vi "Client HTTP Download.vi"(0 "http URL":string, 5 "file path (Not A Path)":path, 7 "follow redirects (T)":bool=TRUE, 9 "Port (80)":u16=80, 11 "error in (no error)":errorcluster) -> (2 "header":string, 3 "status":i32, 4 "full document URL":string, 6 "file path out":path, 8 "file error":errorcluster, 10 "success":bool, 13 "content-type":string, 14 "content":string, 15 "error out":errorcluster)   [LabVIEW 2011]
doc: "Retrieves a document specified by <B>http URL</B> and stores it in a specified file or returns the contents as a string."
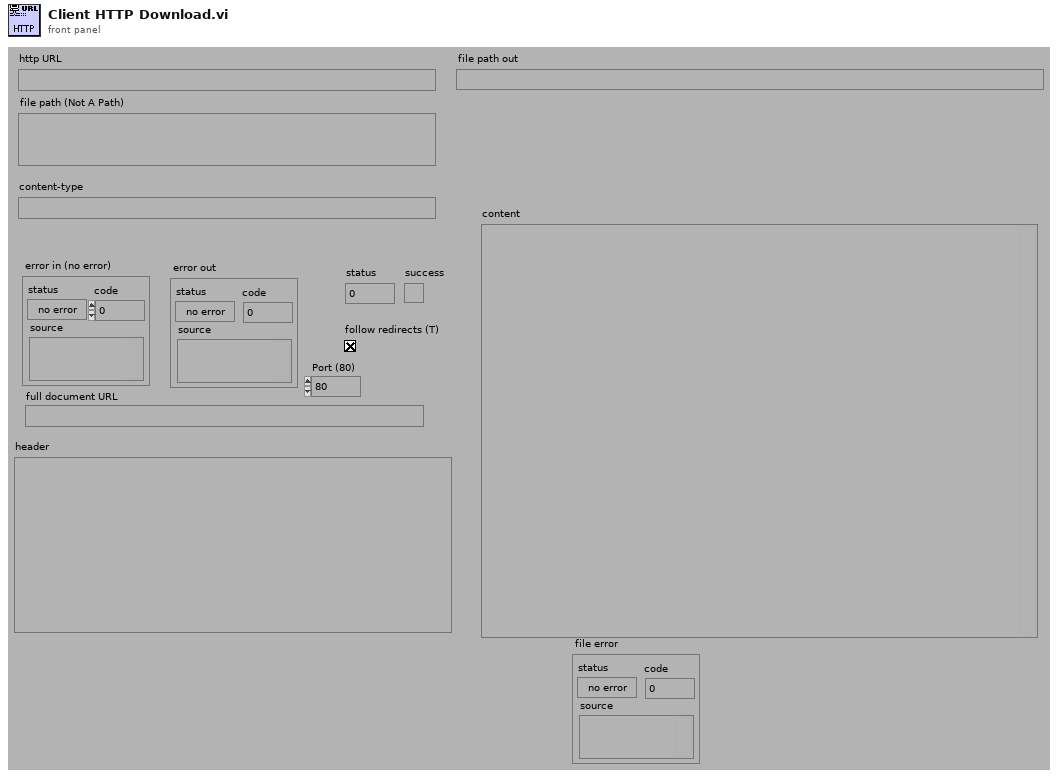
[diagram p1: front panel]
types:
  T1 = cluster{"bytes to read":i32, "timeout ms":i32, "read mode":enum16{"normal", "line", "buffered"}, "line separator":string}
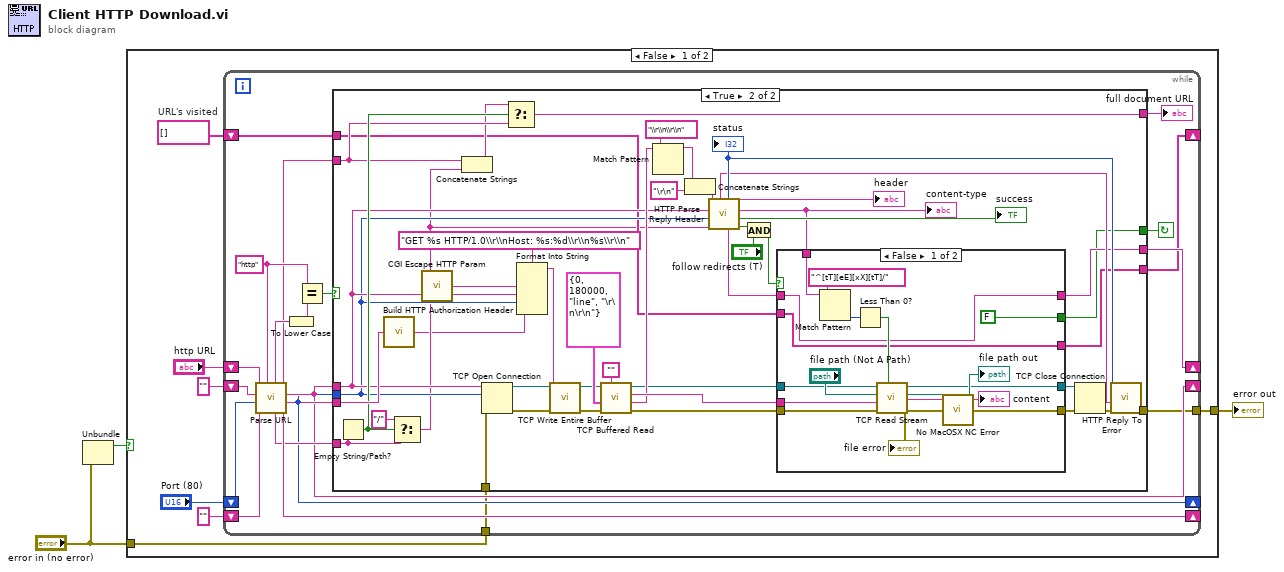
[diagram p0: block diagram]
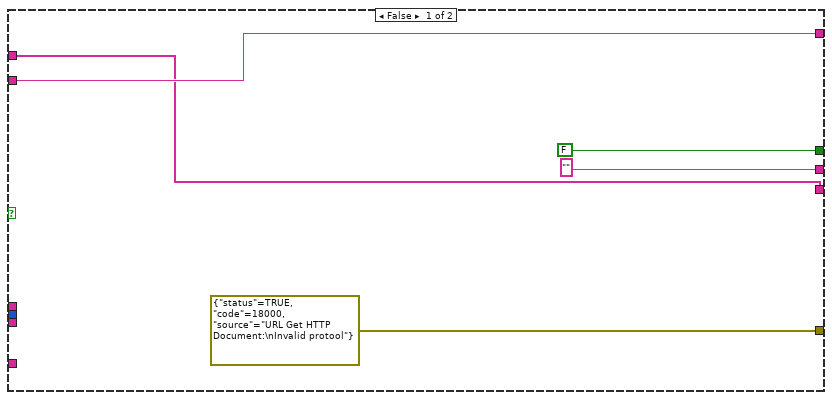
[diagram p2: hidden frame]
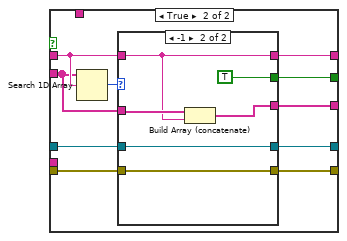
[diagram p3: hidden frame]
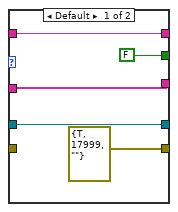
[diagram p4: hidden frame]
diagram:
  n1 = Unbundle("error in (no error)") -> ("status"=w1:bool)  [unwired: 2 out]
  n2 = case shown="False" w1 {
    tunnel: "error in (no error)" -> [w10 w120]
    tunnel: [w9 w120] -> w3
    frame False {
      w4 = string[] []  # URL's visited
      n3 = while {
        tunnel: w10 -> [w18]
        tunnel: [w19] -> w9
        shift-left: "" ("host") -> [w26]
        shift-right: [w24] -> _
        shift-left: "http URL" -> [w28]
        shift-right: [w27] -> _
        shift-left: "Port (80)" -> [w29]
        shift-right: [w20] -> _
        shift-left: "" ("host") -> [w30]
        shift-right: [w21] -> _
        shift-right: [w11] -> _
        shift-left: w4 -> [w12]
        stop <- w25 continue-if-true
        w22 = "http" ("default protocol (\"http\")")
        n4 = call "Parse URL.vi"("default protocol (http)"=w22, "default user:password (none)"=w26, "default port (80)"=w29, "default host"=w30, "URL"=w28) -> ("user:password"=w24:string, "port"=w20:u16, "host"=w21:string, "full URL"=w14:string, "virtual path"=w23:string, "protocol"=w17:string)  [unwired: 1 out]
        n5 = To Lower Case(string=w17) -> (all lower case string=w15:string)
        n6 = Equal?(x=w22, y=w15) -> (x = y?=w16:bool)
        n7 = case shown="True" w16 {
          tunnel: w18 -> [_ w81]
          tunnel: [errorcluster {"status"=TRUE, "code"=18000, "source"="URL Get HTTP Document:\nInvalid protool"} ("error out") w55] -> w19
          tunnel: w20 -> [_ w46]
          tunnel: w21 -> [_ w47]
          tunnel: w23 -> [_ w76]
          tunnel: w24 -> [_ w74]
          tunnel: [FALSE w41] -> w25
          tunnel: ["" ("new location") w43] -> w27
          tunnel: w14 -> [w32 w51]
          tunnel: [w32 w49] -> w13
          tunnel: w12 -> [w31 w45]
          tunnel: [w31 w40] -> w11
          frame False {
          }
          frame True {
            n8 = Empty String/Path?(string/path=w76) -> (empty?=w52:bool)
            n9 = call "Build HTTP Authorization Header.vi"("url authorization"=w74) -> ("HTTP header line"=w36:string)
            n10 = Select(t="/" ("host"), s=w52, f=w76) -> (s? t:f=w38:string)
            n11 = call "CGI Escape HTTP Param.vi"("string"=w38) -> ("url-encoded string"=w37:string)
            n12 = Concatenate Strings(w51, w38) -> (w50:string)
            n13 = TCP Open Connection(address=w47, remote port or service name=w46, error in (no error)=w81) -> (connection ID=w59:refnum<k5>, error out=w60:errorcluster)  [unwired: 2 out]
            n14 = Select(t=w50, s=w52, f=w51) -> (s? t:f=w49:string)
            n15 = Format Into String(format string="GET %s HTTP/1.0\\r\\nHost: %s:%d\\r\\n%s\\r\\n", w37, w47, w46, w36) -> (resulting string=w39:string)  [unwired: 2 in, 1 out]
            n16 = call "TCP Write Entire Buffer.vi"("error in (no error)"=w60, "data in"=w39, "connection ID"=w59) -> ("error out"=w65:errorcluster, "connection ID out"=w61:refnum<k5>)  [unwired: 7 out]
            n17 = call "TCP Buffered Read.vi"("error in (no error)"=w65, "read info"=T1 {"bytes to read"=0, "timeout ms"=180000, "read mode"=enum."line", "line separator"="\r\n\r\n"}, "buffer in"="", "connection ID"=w61) -> ("error out"=w67:errorcluster, "data"=w71:string, "buffer out"=w72:string, "connection ID out"=w68:refnum<k5>)  [unwired: 4 out]
            n18 = Match Pattern(string=w71, regular expression="\\r\\n\\r\\n") -> (before substring=w78:string)  [unwired: 4 out]
            n19 = Concatenate Strings(w78, "\r\n" ("regular expression")) -> (w79:string)
            n20 = call "HTTP Parse Reply Header.vi"("virtual path"=w38, "port"=w46, "host"=w47, "http header"=w79) -> ("redirect?"=w62:bool, "success?"=→"success":bool, "Content-type"=w48:string, "http header out"=→"header":string, "new location"=w44:string, "status"=w54:i32, "status line"=w53:string)  [unwired: 1 out]
            "status" <- w54
            "content-type" <- w48
            n21 = And(x=w62, y="follow redirects (T)") -> (x .and. y?=w42:bool)
            n22 = case shown="False" w42 {
              tunnel: w72 -> [w96 _]
              tunnel: [w94 w101] -> w70
              tunnel: [w83 w99] -> w69
              tunnel: w68 -> [w93 w102]
              tunnel: w67 -> [w92 w100]
              tunnel: w48 -> [w90 _]
              tunnel: w45 -> [w85 w104]
              tunnel: w44 -> [w87 w107]
              tunnel: [w87 w106] -> w43
              tunnel: [FALSE w105] -> w41
              tunnel: [w85 w103] -> w40
              frame False {
                n23 = Match Pattern(string=w90, regular expression="^[tT][eE][xX][tT]/") -> (offset past match=w89:i32)  [unwired: 4 out]
                n24 = Less Than 0?(x=w89) -> (x < 0?=w88:bool)
                n25 = call "TCP Read Stream.vi"("binary"=w88, "error in (no error)"=w92, "header (\"\")"=w96, "data file (<NAP>)"="file path (Not A Path)", "connection"=w93) -> ("error out"=w84:errorcluster, "data"=→"content":string, "data file out"=→"file path out":path, "duplicate connection"=w94:refnum<k5>, "file error"=→"file error":errorcluster)  [unwired: 2 in]
                n26 = call "No MacOSX NC Error.vi"("error in (no error)"=w84) -> ("error out"=w83:errorcluster)  [unwired: 4 out]
              }
              frame True {
                n27 = Search 1D Array(1D array=w104, element=w107) -> (index of element=w108:i32)  [unwired: 1 out]
                n28 = case shown="-1" w108 {
                  tunnel: w107 -> [w110 w117]
                  tunnel: [w110 w117] -> w106
                  tunnel: [FALSE TRUE] -> w105
                  tunnel: w104 -> [w112 w118]
                  tunnel: [w112 w116] -> w103
                  tunnel: w102 -> [w113 w115]
                  tunnel: [w113 w115] -> w101
                  tunnel: w100 -> [_ w114]
                  tunnel: [errorcluster {"status"=TRUE, "code"=17999, "source"=""} ("error out") w114] -> w99
                  frame Default {
                  }
                  frame -1 {
                    n29 = Build Array (concatenate)(w118, w117) -> (w116:string[])
                  }
                }
              }
            }
            n30 = TCP Close Connection(connection ID=w70, error in (no error)=w69) -> (error out=w56:errorcluster)  [unwired: 2 out]
            n31 = call "HTTP Reply To Error.vi"("error in (no error)"=w56, "reply string in"=w53, "reply code in"=w54) -> ("error out"=w55:errorcluster)  [unwired: 4 out]
          }
        }
        "full document URL" <- w13
      }
    }
    frame True {
    }
  }
  "error out" <- w3
